vi "Stepper_Sub_New.vi"(6 "First Motor Pin":u8=3, 8 "error in":errorcluster, 9 "Direction":bool=TRUE, 10 "Velocity":dbl, 11 "Arduino Resource":T1={"VISA resource"="COM10", "Board Type"=enum."Mega 2560", "Connection Type"=enum."USB / Serial", "Bytes Per Packet (15)"=15}) -> (0 "error out":errorcluster={"status"=FALSE, "code"=1073676294, "source"="VISA Read in LabVIEW Interface for Arduino.lvlib:Send Receive.vi->Stepper_Sub.vi"}, 3 "Arduino Resource 2":T1={"VISA resource"="COM10", "Board Type"=enum."Mega 2560", "Connection Type"=enum."USB / Serial", "Bytes Per Packet (15)"=15})   [LabVIEW 2013]
uses:
  <vilib>/LabVIEW Interface for Arduino/Type Defs/Arduino Resource.ctl
  <vilib>/LabVIEW Interface for Arduino/Type Defs/Board Type.ctl
  <vilib>/LabVIEW Interface for Arduino/Type Defs/Pin Mode.ctl
  <vilib>/LabVIEW Interface for Arduino/LabVIEW Interface for Arduino.lvlib
panel:
  out "x+1":u8
  out "Current Output":bool[](array[boolean])=[FALSE, FALSE, FALSE, TRUE]
  in  "Stepper Pattern":bool[][](array[boolean])=[[TRUE, FALSE, FALSE, TRUE, TRUE, FALSE, FALSE, FALSE], [FALSE, TRUE, TRUE, FALSE, FALSE, TRUE, TRUE, FALSE], [TRUE, TRUE, FALSE, FALSE, TRUE, TRUE, FALSE, FALSE], [FALSE, FALSE, TRUE, TRUE, FALSE, FALSE, TRUE, TRUE], [FALSE, FALSE, FALSE, FALSE, FALSE, FALSE, FALSE, FALSE], [FALSE, FALSE, FALSE, FALSE, FALSE, FALSE, FALSE, FALSE], [FALSE, FALSE, FALSE, FALSE, FALSE, FALSE, FALSE, FALSE], [FALSE, FALSE, FALSE, FALSE, FALSE, FALSE, FALSE, FALSE]]
  out "sequence":i32=7
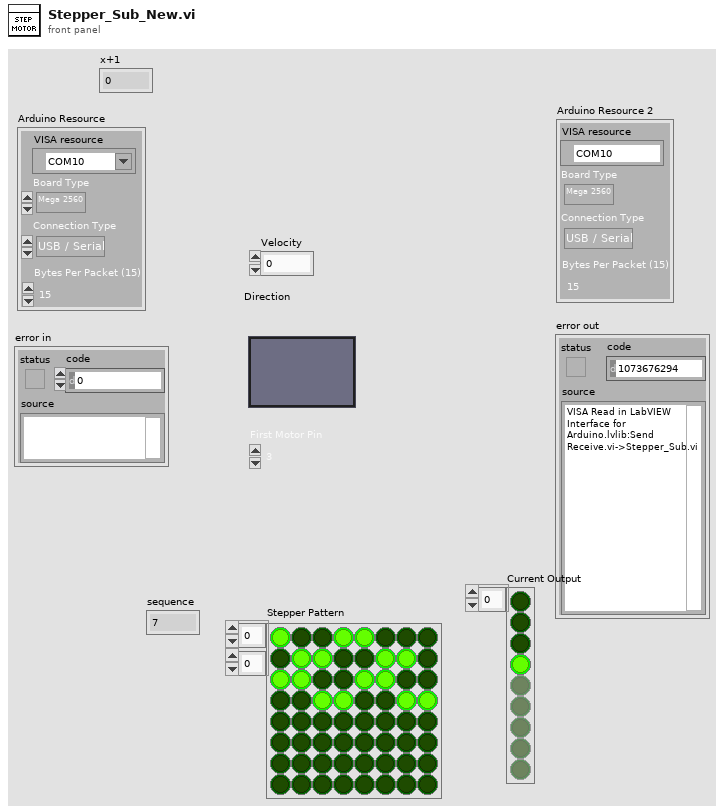
[diagram p1: front panel]
types:
  T1 = typedef "LabVIEW Interface for Arduino.lvlib/Arduino Resource.ctl" = cluster{"VISA resource":refnum<visa-resource-name>, "Board Type":T2, "Connection Type":enum8{"USB / Serial"}, "Bytes Per Packet (15)":u8}
  T2 = typedef "LabVIEW Interface for Arduino.lvlib/Board Type.ctl" = enum16{"Uno", "Dimuelanove w/Atmega 328", "Mega 2560"}
  T3 = typedef "LabVIEW Interface for Arduino.lvlib/Pin Mode.ctl" = enum8{"Input", "Output"}
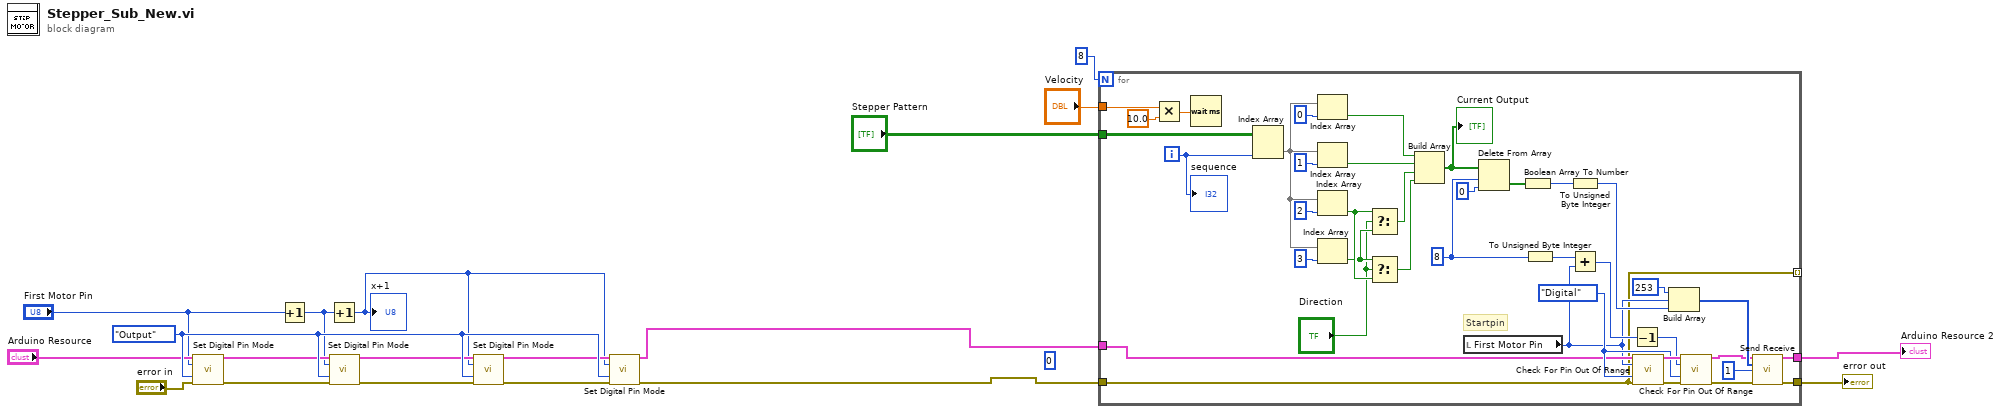
[diagram p0: block diagram]
diagram:
  (unwired) u8 0 ("x")
  w19 = Pin_Mode."Output" ("Pin Mode (Input)")
  n1 = call <vilib>:"Set Digital Pin Mode.vi"("Arduino Resource"="Arduino Resource", "Digital I/O Pin"="First Motor Pin", "Pin Mode (Input)"=w19, "error in"="error in") -> ("Arduino Resource"=w18:T1, "error out"=w15:errorcluster)  [unwired: 10 in]
  n2 = Increment(x="First Motor Pin") -> (x+1=w8:u8)
  n3 = Increment(x=w8) -> (x+1=w5:u8)
  "x+1" <- w5
  n4 = call <vilib>:"Set Digital Pin Mode.vi"("Arduino Resource"=w18, "Digital I/O Pin"=w8, "Pin Mode (Input)"=w19, "error in"=w15) -> ("Arduino Resource"=w17:T1, "error out"=w14:errorcluster)  [unwired: 10 in]
  n5 = call <vilib>:"Set Digital Pin Mode.vi"("Arduino Resource"=w17, "Digital I/O Pin"=w5, "Pin Mode (Input)"=w19, "error in"=w14) -> ("Arduino Resource"=w16:T1, "error out"=w13:errorcluster)  [unwired: 10 in]
  n6 = call <vilib>:"Set Digital Pin Mode.vi"("Arduino Resource"=w16, "Digital I/O Pin"=w5, "Pin Mode (Input)"=w19, "error in"=w13) -> ("Arduino Resource"=w3:T1, "error out"=w4:errorcluster)  [unwired: 10 in]
  n7 = for {
    N: 8 -> [_]
    tunnel: "Stepper Pattern" -> [w57]
    tunnel: "Velocity" -> [w49]
    tunnel: w3 -> [w31]
    tunnel: [w20] -> _ mode=indexing
    tunnel: [w30] -> w7
    tunnel: [w29] -> w6
    tunnel: w4 -> [w20]
    i -> [w58]
    w37 = enum16{"Analog", "Digital"}."Digital" ("Pin Type")
    w35 = 8 ("length")
    # "Startpin"
    n8 = Multiply(x=w49, y=10.0) -> (x*y=w50:dbl)
    n9 = Wait (ms)(milliseconds to wait=w50) -> ()  [unwired: 1 out]
    n10 = Index Array(array=w57, index (col)=w58) -> (element=w27:bool[])  [unwired: 1 in]
    n11 = Index Array(array=w27, index=0) -> (element=w21:bool)
    n12 = Index Array(array=w27, index=1) -> (element=w22:bool)
    n13 = Index Array(array=w27, index=2) -> (element=w26:bool)
    n14 = Index Array(array=w27, index=3) -> (element=w25:bool)
    n15 = Select(t=w26, s="Direction", f=w25) -> (s? t:f=w52:bool)
    n16 = Select(t=w25, s="Direction", f=w26) -> (s? t:f=w51:bool)
    n17 = Build Array(w21, w22, w52, w51) -> (w23:bool[])
    "Current Output" <- w23
    n18 = local read "First Motor Pin"() -> (w28:u8)
    n19 = Delete From Array(array=w23, length=w35, index=0) -> (deleted portion=w43:bool[])  [unwired: 1 out]
    n20 = Boolean Array To Number(Boolean array=w43) -> (number=w44:u32)
    n21 = To Unsigned Byte Integer(number=w35) -> (unsigned 8bit integer=w34:u8)
    n22 = To Unsigned Byte Integer(number=w44) -> (unsigned 8bit integer=w32:u8)
    n23 = Add(x=w34, y=w28) -> (x+y=w36:u8)
    n24 = Decrement(x=w36) -> (x-1=w33:u8)
    n25 = call <vilib>:"Check For Pin Out Of Range.vi"("Arduino Resource"=w31, "User Pin Number"=w28, "Pin Type"=w37, "error in"=w20) -> ("Arduino Resource"=w41:T1, "error out"=w40:errorcluster)  [unwired: 10 in]
    n26 = Build Array(u8 253, w28, w32) -> (w47:u8[])
    n27 = call <vilib>:"Check For Pin Out Of Range.vi"("Arduino Resource"=w41, "User Pin Number"=w33, "Pin Type"=w37, "error in"=w40) -> ("Arduino Resource"=w38:T1, "error out"=w39:errorcluster)  [unwired: 10 in]
    n28 = call <vilib>:"Send Receive.vi"("Arduino Resource"=w38, "Data"=w47, "Bytes To Read (0)"=u32 1, "error in"=w39) -> ("Arduino Resource"=w30:T1, "error out"=w29:errorcluster)  [unwired: 9 in, 1 out]
    "sequence" <- w58
  }
  "error out" <- w6
  "Arduino Resource 2" <- w7
